vi "写入固件.vi"(8 "错误输入":errorcluster, 10 "保留原配置":bool=TRUE, 11 "MB session in":refnum<class "MB_Master.lvclass">) -> (0 "error out":errorcluster, 3 "MB session out":refnum<class "MB_Master.lvclass">)   [LabVIEW 2016, in "斯坦道CODMn新电路板.lvlib"]
uses:
  <vilib>/Plasmionique/MB Master/MB_Master/MB_Master.lvclass
  <vilib>/NI/Progress Bar/Controls/Update Bar Actions.ctl
  <vilib>/NI/Progress Bar/Controls/Progress Bar Properties.ctl
  <vilib>/Plasmionique/MB Master/MB_Master_Serial/MB_Master_Serial.lvclass
  D:/Program Files (x86)/National Instruments/LabVIEW 2016/vi.lib/Plasmionique/MB Master/MB_Master/MB_Master.lvclass
  <vilib>/regexp/Match Regular Expression.xnode
  <vilib>/Plasmionique/MB Master/MB Master.lvlib
  <vilib>/NI/Progress Bar/Progress Bar.lvlib
panel:
  in  "引用选择":enum16{"MB引用", "自建引用"}(ring)
  in  "VISA Resource":refnum<visa-resource-name>
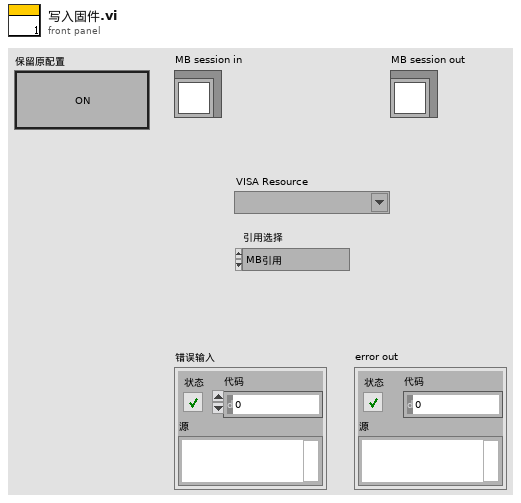
[diagram p1: front panel]
types:
  T1 = enum16{"open", "replace", "create", "open or create", "replace or create", "replace or create with confirmation"}
  T2 = enum16{"big-endian, network order", "native, host order", "little-endian"}
  T3 = typedef "Progress Bar.lvlib/Update Bar Actions.ctl" = enum16{"Add To Existing", "Set to Value"}
  T4 = cluster{"baud rate (bps)":u32, "stop bits":u16, "parity":u16, "flow control":u16, "timeout":u32, "retries":i32}
  T5 = typedef "Progress Bar.lvlib/Progress Bar Properties.ctl" = cluster{"Background Color":u32, "Installer Title":string, "Title Color":u32, "Action Text":string, "Text Color":u32, "Slider Value":u8, "Bar Color":u32, "Timeout":i32}
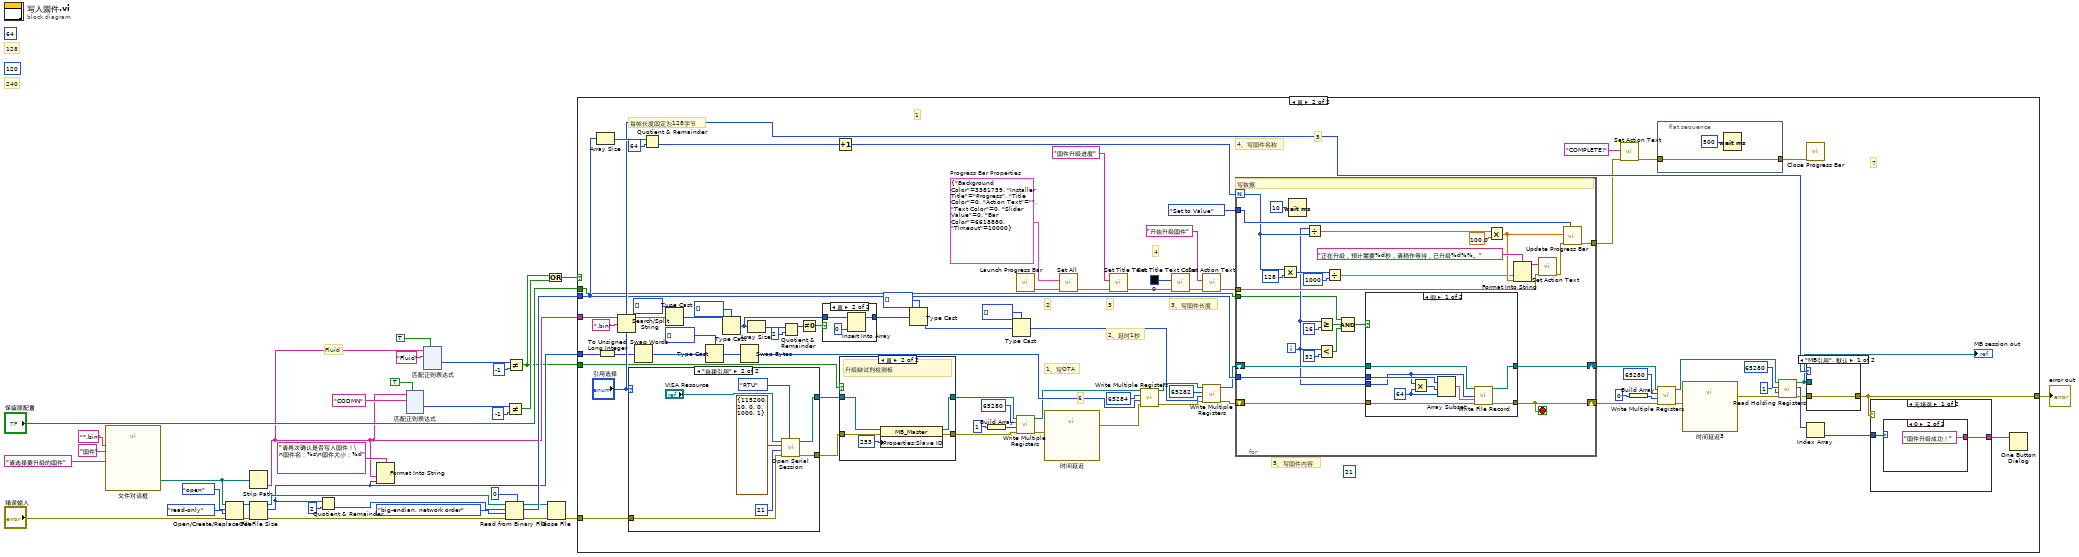
[diagram p0: block diagram]
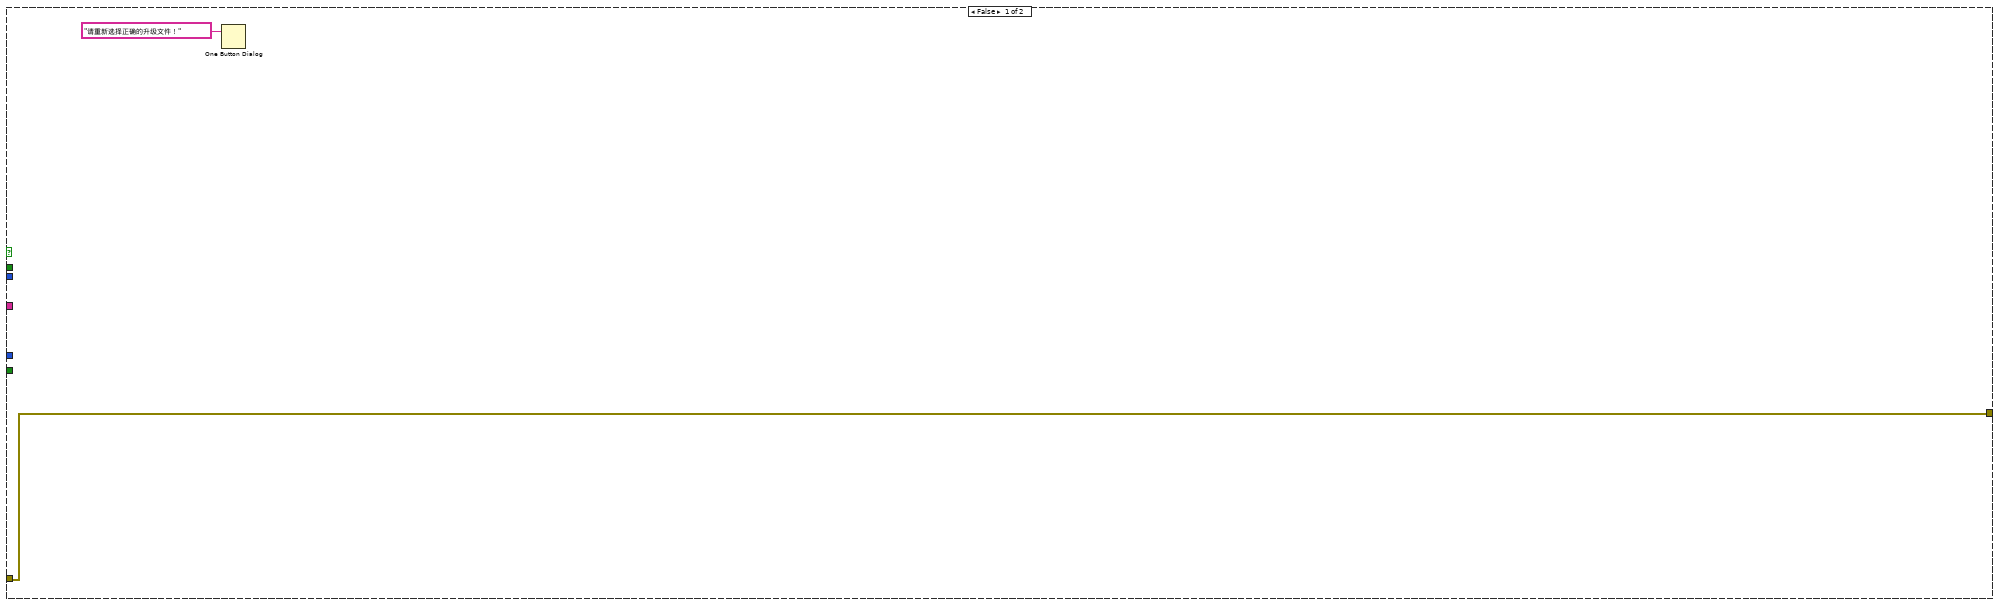
[diagram p2: hidden frame]
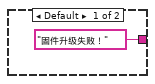
[diagram p5: hidden frame]
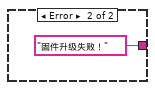
[diagram p6: hidden frame]
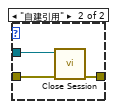
[diagram p7: hidden frame]
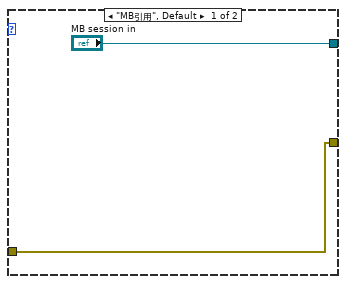
[diagram p8: hidden frame]
diagram:
  (unwired) 64 ("y")
  (unwired) 120 ("y")
  # "Fluid"
  # "240"
  # "128"
  n1 = call "文件对话框"("prompt"="请选择要升级的固件", "pattern (all files)"="*.bin", "pattern label"="固件") -> ("selected path"=w26:path)  [unwired: 9 in, 3 out]
  n2 = Open/Create/Replace File(file path (use dialog)=w26, error in="错误输入", operation (0:open)=T1."open" ("操作(0:open)"), access (0:read/write)=enum16{"read/write", "read-only", "write-only"}."read-only" ("权限(0:read/write)")) -> (refnum out=w25:refnum<file>, error out=w23:errorcluster)  [unwired: 2 in, 1 out]
  n3 = Strip Path(path=w26) -> (name=w3:string)  [unwired: 1 out]
  n4 = Get File Size(file=w25, error in=w23) -> (refnum out=w24:refnum<file>, size (in bytes)=w18:i64, 0:w22:errorcluster)
  n5 = Quotient & Remainder(x=w18, y=i64 2) -> (floor(x/y)=w20:i64)  [unwired: 1 out]
  n6 = Format Into String(format string="请再次确认是否写入固件！\n固件名：%s\n固件大小：%d" ("格式字符串"), w3, w18) -> ()  [unwired: 2 in, 2 out]
  n7 = xnode "匹配正则表达式"("输入字符串"=w3, "正则表达式"="CODMN", "忽略大小写？(F)"=TRUE) -> ("匹配后偏移量"=w13:i32)  [unwired: 3 in, 4 out]
  n8 = xnode "匹配正则表达式"("输入字符串"=w3, "正则表达式"="Fluid", "忽略大小写？(F)"=TRUE) -> ("匹配后偏移量"=w6:i32)  [unwired: 3 in, 4 out]
  n9 = Read from Binary File(5:u16 0, 8:w22, 9:T2."big-endian, network order" ("字节顺序(0:big-endian, network order)"), 10:w20, 11:w24) -> (0:w10:errorcluster, 2:w19:u16[], 3:w11:refnum<file>)  [unwired: 1 in, 1 out]
  n10 = Not Equal?(x=w13, y=-1) -> (x != y?=w8:bool)
  n11 = Not Equal?(x=w6, y=-1) -> (x != y?=w1:bool)
  n12 = Or(x=w1, y=w8) -> (x .or. y?=w2:bool)
  n13 = Close File(refnum=w11, error in=w10) -> (error out=w9:errorcluster)  [unwired: 1 out]
  n14 = case shown="真" w2 {
    tunnel: w19 -> [_ w83]
    tunnel: w3 -> [_ w98]
    tunnel: w9 -> [w37 w99]
    tunnel: [w37 w80] -> w29
    tunnel: w18 -> [_ w85]
    tunnel: "保留原配置" -> [_ w53]
    tunnel: w1 -> [_ w50]
    frame False {
      n15 = One Button Dialog(message="请重新选择正确的升级文件！" ("消息")) -> ()  [unwired: 1 in, 1 out]
    }
    frame True {
      w77 = T5 {"Background Color"=3381759, "Installer Title"="Progress", "Title Color"=0, "Action Text"="", "Text Color"=0, "Slider Value"=0, "Bar Color"=6618880, "Timeout"=10000}  # Progress Bar Properties
      (unwired) 21 ("Value")
      # "7"
      # "6"
      # "5"
      # "4"
      # "3"
      # "2"
      # "1"
      # "每帧长度固定为128字节"
      # "5、写固件内容"
      # "4、写固件名称"
      # "3、写固件长度"
      # "2、延时1秒"
      # "1、写OTA"
      n16 = Array Size(array=w83) -> (size(s)=w113:i32)
      n17 = To Unsigned Long Integer(number=w85) -> (unsigned 32bit integer=w82:u32)
      n18 = Search/Split String(string=w98, search string/char (-)=".bin" ("搜索字符串/字符(-)")) -> (substring before match=w96:string)  [unwired: 1 in, 2 out]
      n19 = case shown="\"自建引用\"" "引用选择" {
        tunnel: ["MB session in" w144] -> w52
        tunnel: w99 -> [w138 w143]
        tunnel: [w138 w142] -> w49
        frame "MB引用", Default {
        }
        frame "自建引用" {
          n20 = call <vilib>:"Open Serial Session.vi"("Mode (RTU)"=enum16{"RTU", "ASCII"}."RTU", "Error in"=w143, "Slave ID"=u8 21, "Serial Config"=T4 {"baud rate (bps)"=115200, "stop bits"=10, "parity"=0, "flow control"=0, "timeout"=1000, "retries"=1}, "VISA Resource"="VISA Resource") -> ("Error out"=w142:errorcluster, "MB_Serial session"=w144:refnum<class "MB_Master_Serial.lvclass">)  [unwired: 5 in]
        }
      }
      n21 = Swap Words(1:w82) -> (0:w81:u32)
      n22 = Quotient & Remainder(x=w113, y=64) -> (floor(x/y)=w114:i32)  [unwired: 1 out]
      n23 = Type Cast(type=u8[] [], x=w96) -> (*(type *) &x=w39:u8[])
      n24 = Type Cast(type=u16[] [], x=w81) -> (*(type *) &x=w107:u16[])
      n25 = Type Cast(type=u8[] [], x=w39) -> (*(type *) &x=w40:u8[])
      n26 = Swap Bytes(anything=w107) -> (byte swapped=w106:u16[])
      n27 = Array Size(array=w40) -> (size(s)=w41:i32)
      n28 = Quotient & Remainder(x=w41, y=2) -> (x-y*floor(x/y)=w43:i32)  [unwired: 1 out]
      n29 = Not Equal To 0?(x=w43) -> (x != 0?=w42:bool)
      n30 = case shown="真" w42 {
        tunnel: w40 -> [w115 w117]
        tunnel: [w115 w116] -> w45
        frame False {
        }
        frame True {
          n31 = Insert Into Array(array=w117, new element=u8 0 ("新元素/子数组")) -> (w116:u8[])  [unwired: 1 in]
        }
      }
      n32 = Increment(x=w114) -> (x+1=w84:i32)
      n33 = case shown="真" w50 {
        tunnel: w52 -> [w120 w125]
        tunnel: [w120 w124] -> w51
        tunnel: w49 -> [w119 w121]
        tunnel: [w119 w122] -> w48
        frame False {
          # "升级主板"
        }
        frame True {
          # "升级缺试剂检测板"
          n34 = property class="MB_Master"(reference=w125, error in=w121, "Properties:Slave ID"=u8 253 ("Slave ID")) -> (reference out=w124:refnum<class "MB_Master.lvclass">, error out=w122:errorcluster)
        }
      }
      n35 = Type Cast(type=u16[] [], x=w45) -> (*(type *) &x=w38:u16[])
      n36 = Build Array(u16 1 ("value")) -> (w100:u16[])
      n37 = Type Cast(type=u16[] [], x=w38) -> (*(type *) &x=w95:u16[])
      n38 = call <vilib>:"Launch Progress Bar.vi"() -> ("error out"=w76:errorcluster)  [unwired: 10 in, 1 out]
      n39 = call <vilib>:"Write Multiple Registers.vi"("error in (no error)"=w48, "values"=w100, "starting address"=u16 65280, "MB session in"=w51) -> ("error out"=w109:errorcluster, "MB session out"=w88:refnum<class "MB_Master.lvclass">)  [unwired: 6 in]
      n40 = call "时间延迟"("error in (no error)"=w109) -> ("error out"=w89:errorcluster)  [unwired: 10 in]
      n41 = call <vilib>:"Set All.vi"("error in (no error)"=w76, "Progress Bar Properties (Default)"=w77) -> ("error out"=w70:errorcluster)  [unwired: 9 in]
      n42 = call <vilib>:"Set Title Text.vi"("error in (no error)"=w70, "Installer Title"="固件升级进度") -> ("error out"=w68:errorcluster)  [unwired: 9 in]
      n43 = call <vilib>:"Write Multiple Registers.vi"("error in (no error)"=w89, "values"=w106, "starting address"=u16 65284, "MB session in"=w88) -> ("error out"=w104:errorcluster, "MB session out"=w105:refnum<class "MB_Master.lvclass">)  [unwired: 6 in]
      n44 = call <vilib>:"Set Title Text Color.vi"("error in (no error)"=w68, "Color Box"=u32 0) -> ("error out"=w71:errorcluster)  [unwired: 9 in]
      n45 = call <vilib>:"Set Action Text.vi"("error in (no error)"=w71, "Action Text"="开始升级固件") -> ("error out"=w65:errorcluster)  [unwired: 9 in]
      n46 = call <vilib>:"Write Multiple Registers.vi"("error in (no error)"=w104, "values"=w95, "starting address"=u16 65282, "MB session in"=w105) -> ("error out"=w62:errorcluster, "MB session out"=w63:refnum<class "MB_Master.lvclass">)  [unwired: 6 in]
      n47 = for {
        N: w84 -> [w155]
        shift-right: [w170] -> w58
        shift-left: w63 -> [w172]
        shift-right: [w146] -> w54
        shift-left: w62 -> [w171]
        tunnel: w83 -> [w168]
        tunnel: Update_Bar_Actions."Set to Value" ("Action") -> [w167]
        tunnel: w65 -> [w165]
        tunnel: [w166] -> w64
        tunnel: w53 -> [w147]
        i -> [w152]
        stop <- w146 stop-if-true
        # "写数据"
        n48 = Multiply(x=w155, y=128) -> (x*y=w159:i32)
        n49 = Wait (ms)(milliseconds to wait=u32 10) -> ()  [unwired: 1 out]
        n50 = Divide(x=w152, y=w155) -> (x/y=w161:dbl)
        n51 = Greater Or Equal?(x=w152, y=16) -> (x >= y?=w150:bool)
        n52 = Less?(x=w152, y=32) -> (x < y?=w149:bool)
        n53 = Divide(x=w159, y=u32 1000) -> (x/y=w156:dbl)
        n54 = Compound Arithmetic op=AND ("复合运算")(w147, w150, w149) -> (w148:bool)
        n55 = case shown="假" w148 {
          tunnel: w172 -> [w181 w183]
          tunnel: w171 -> [w180 w182]
          tunnel: [w179 w183] -> w170
          tunnel: [w178 w182] -> w146
          tunnel: w168 -> [w177 _]
          tunnel: w152 -> [w173 _]
          frame False {
            w175 = 64 ("长度")
            n56 = Multiply(x=w173, y=w175) -> (x*y=w174:i32)
            n57 = Array Subset(array=w177, index=w174, length=w175) -> (w176:u16[])
            n58 = call "Write File Record.vi"("MB session in"=w181, "Record Number"=w173, "values"=w176, "error in (no error)"=w180) -> ("MB session out"=w179:refnum<class "MB_Master.lvclass">, "error out"=w178:errorcluster)  [unwired: 10 in]
          }
          frame True {
            # "保留原配置"
          }
        }
        n59 = Multiply(x=w161, y=100.0) -> (x*y=w157:dbl)
        n60 = Format Into String(format string="正在升级，预计需要%d秒，请稍作等待，已升级%d%%。" ("格式字符串"), w156, w157) -> (resulting string=w162:string)  [unwired: 2 in, 1 out]
        n61 = call <vilib>:"Set Action Text.vi"("error in (no error)"=w165, "Action Text"=w162) -> ("error out"=w164:errorcluster)  [unwired: 9 in]
        n62 = call <vilib>:"Update Progress Bar.vi"("Action"=w167, "error in (no error)"=w164, "Value"=w157) -> ("error out"=w166:errorcluster)  [unwired: 8 in]
      }
      n63 = call <vilib>:"Set Action Text.vi"("error in (no error)"=w64, "Action Text"="COMPLETE!") -> ("error out"=w73:errorcluster)  [unwired: 9 in]
      n64 = Build Array(0 ("value")) -> (w59:i32[])
      n65 = flat-sequence {
        tunnel: w73 -> [w126]
        tunnel: [w126] -> w75
        frame #0 {
          n66 = Wait (ms)(milliseconds to wait=u32 500) -> ()  [unwired: 1 out]
        }
      }
      n67 = call <vilib>:"Write Multiple Registers.vi"("error in (no error)"=w54, "values"=w59, "starting address"=u16 65280, "MB session in"=w58) -> ("error out"=w56:errorcluster, "MB session out"=w57:refnum<class "MB_Master.lvclass">)  [unwired: 6 in]
      n68 = call "时间延迟3"("error in (no error)"=w56) -> ("error out"=w55:errorcluster)  [unwired: 10 in]
      n69 = call <vilib>:"Read Holding Registers.vi"("error in (no error)"=w55, "quantity"=u16 1, "starting address"=u16 65280, "MB session in"=w57) -> ("error out"=w86:errorcluster, "Registers"=w90:u16[], "MB session out"=w87:refnum<class "MB_Master.lvclass">)  [unwired: 5 in]
      "MB session out" <- w87
      n70 = call <vilib>:"Close Progress Bar.vi"("error in (no error)"=w75) -> ()  [unwired: 9 in, 2 out]
      n71 = case shown="\"MB引用\", 默认" "引用选择" {
        tunnel: w87 -> [_ w136]
        tunnel: w86 -> [w133 w135]
        tunnel: [w133 w134] -> w80
        frame "MB引用", Default {
        }
        frame "自建引用" {
          n72 = call-dynamic "Close Session.vi"("error in (no error)"=w135, "MB session in"=w136) -> ("error out"=w134:errorcluster)  [unwired: 9 in]
        }
      }
      n73 = Index Array(array=w90) -> (element=w79:u16)  [unwired: 1 in]
      n74 = case shown="无错误" w80 {
        tunnel: w79 -> [w129 _]
        tunnel: [w128 "固件升级失败！"] -> w78
        frame No Error {
          n75 = case shown="0" w129 {
            tunnel: ["固件升级失败！" "固件升级成功！"] -> w128
            frame Default {
            }
            frame 0 {
            }
          }
        }
        frame Error {
        }
      }
      n76 = One Button Dialog(message=w78) -> ()  [unwired: 1 in, 1 out]
    }
  }
  "error out" <- w29
